vi "RollingDice-WithSubVI.vi"() -> ()   [LabVIEW 2018]
panel:
  out "You Win":bool
  out "You Lose":bool
  out "Sum":dbl
  in  "Roll Dice":bool
  out "Dice 2":dbl
  out "Dice 1":dbl
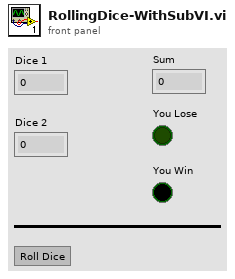
[diagram p1: front panel]
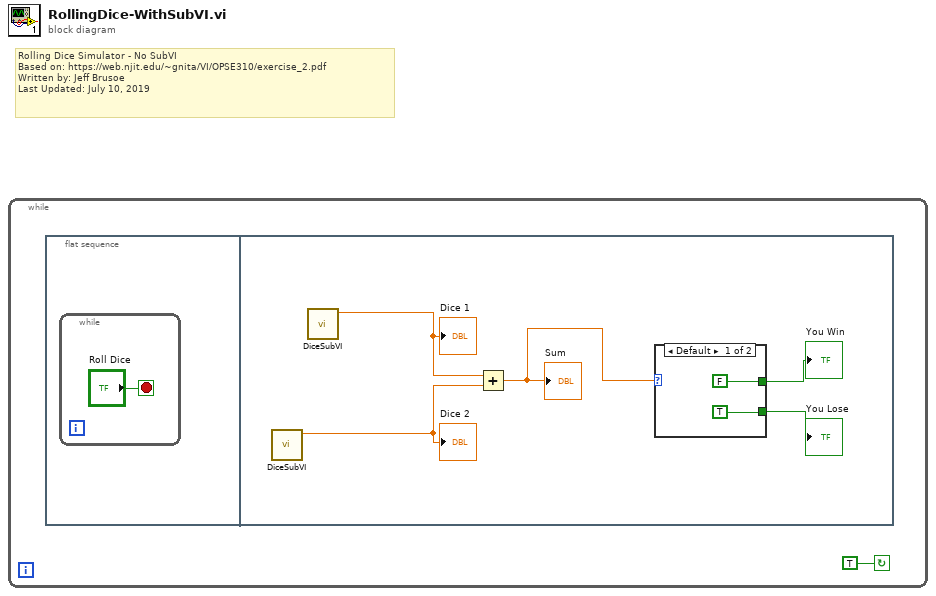
[diagram p0: block diagram]
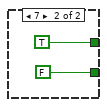
[diagram p2: hidden frame]
diagram:
  # "Rolling Dice Simulator - No SubVI\nBased on: https://web.njit.edu/~gnita/VI/OPSE310/exercise_2.pdf\nWritten by: Jeff Brusoe\nLast Updated: July 10, 2019"
  n1 = while {
    stop <- TRUE continue-if-true
    n2 = flat-sequence {
      frame #0 {
        n3 = while {
          stop <- "Roll Dice" stop-if-true
        }
      }
      frame #1 {
        n4 = call "DiceSubVI.vi"() -> ("Numeric"=w3:dbl)  [unwired: 11 in]
        "Dice 2" <- w3
        n5 = call "DiceSubVI.vi"() -> ("Numeric"=w7:dbl)  [unwired: 11 in]
        "Dice 1" <- w7
        n6 = Add(x=w7, y=w3) -> (x+y=w6:dbl)
        "Sum" <- w6
        n7 = case shown="Default" w6 {
          tunnel: [FALSE TRUE] -> w5
          tunnel: [TRUE FALSE] -> w4
          frame Default {
          }
          frame 7 {
          }
        }
        "You Win" <- w5
        "You Lose" <- w4
      }
    }
  }
